vi "MTM2_logEvent_inclinationTelemetrySource.vi"(8 "error in (no error)":errorcluster, 11 "logevent_inclinationTelemetrySource_Ctl":T1) -> (0 "error out":errorcluster, 2 "function return":i32, 3 "logevent_inclinationTelemetrySource_Ctl out":T1)   [LabVIEW 2018, in "SALLV_MTM2.lvlib"]
doc: "int MTM2_shm_logEvent_inclinationTelemetrySourceLV(MTM2_logevent_inclinationTelemetrySourceLV *logevent_inclinationTelemetrySource_Ctl );"
uses:
  DataTypes/logevent_inclinationTelemetrySource.ctl
  SALLV_MTM2.lvlib
  SALLV_MTM2.so
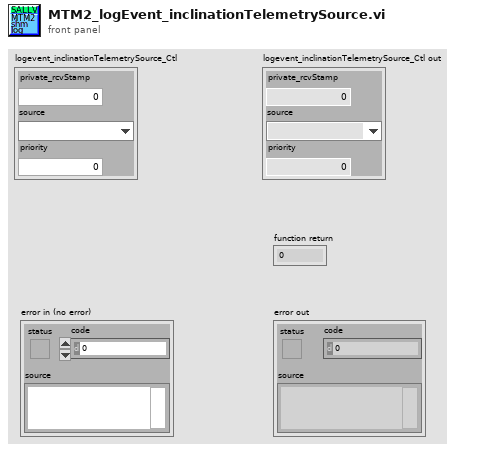
[diagram p1: front panel]
types:
  T1 = typedef "SALLV_MTM2.lvlib/logevent_inclinationTelemetrySource.ctl" = cluster{"private_rcvStamp":dbl, "source":enum32{"", "OnBoard", "MTMount"}, "priority":i32}
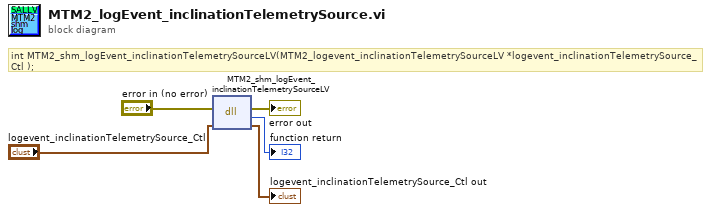
[diagram p0: block diagram]
diagram:
  # "int MTM2_shm_logEvent_inclinationTelemetrySourceLV(MTM2_logevent_inclinationTelemetrySourceLV *logevent_inclinationTelemetrySource_Ctl );"
  n1 = dll-call lib="home/ttsai/Documents/salLabviewApi/SALLV_MTM2/SALLV_MTM2.*" fn="MTM2_shm_logEvent_inclinationTelemetrySourceLV"(error in="error in (no error)", "logevent_inclinationTelemetrySource_Ctl"="logevent_inclinationTelemetrySource_Ctl") -> (error out=→"error out":errorcluster, →"function return":i32, "logevent_inclinationTelemetrySource_Ctl"=→"logevent_inclinationTelemetrySource_Ctl out":T1)  [unwired: 2 in, 1 out]
